vi "setSlitWidth.vi"(8 "error in (no error)":errorcluster, 10 "position":T1, 11 "Monochromator in":refnum<class "Monochromator.lvclass">) -> (0 "error out":errorcluster, 3 "Monochromator out":refnum<class "Monochromator.lvclass">)   [LabVIEW 2020, in "Monochromator.lvclass"]
uses:
  Monochromator.lvclass
  Typedefs/slit.ctl
  Typedefs/SlitType.ctl
  Typedefs/slitWidth.ctl
  Monochromator.lvclass/Monochromator.ctl
  MonoStates/MonoState/MonoState.lvclass
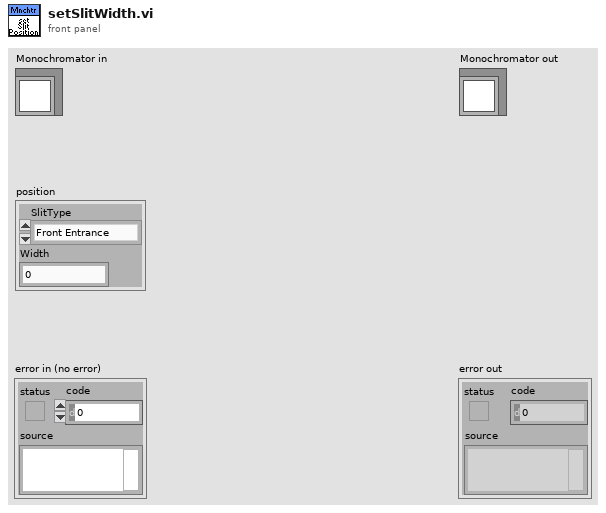
[diagram p1: front panel]
types:
  T1 = typedef "slit.ctl" = cluster{"SlitType":T2, "Width":T3}
  T2 = typedef "SlitType.ctl" = enum16{"Front Entrance", "Side Entrance", "Front Exit", "Side Exit", "First Intermediate", "Second Intermediate"}
  T3 = typedef "slitWidth.ctl" = dbl
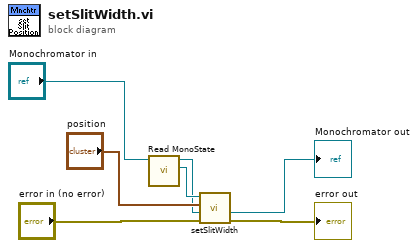
[diagram p0: block diagram]
diagram:
  n1 = call "Read MonoState.vi"("Monochromator in"="Monochromator in") -> ("MonoState.lvclass"=w2:refnum<class "MonoState.lvclass">, "Monochromator out"=w1:refnum<class "Monochromator.lvclass">)  [unwired: 8 in, 1 out]
  n2 = call-dynamic "setSlitWidth.vi"("error in (no error)"="error in (no error)", "Monochromator in"=w1, "position"="position", "MonoState in"=w2) -> ("error out"=→"error out":errorcluster, "Monochromator out"=→"Monochromator out":refnum<class "Monochromator.lvclass">)  [unwired: 5 in, 1 out]
